vi "Ring下拉列表鼠标滚动事件.vi"(8 "error in (no error)":errorcluster caption="错误输入（无错误）", 9 "方向":enum16{"Horizontal", "Vertical"}(ring), 10 "Delta":i32, 11 "CtlRef":refnum<vi>) -> (0 "error out":errorcluster caption="错误输出", 3 "CtlRef 2":refnum<vi>)   [LabVIEW 2018]
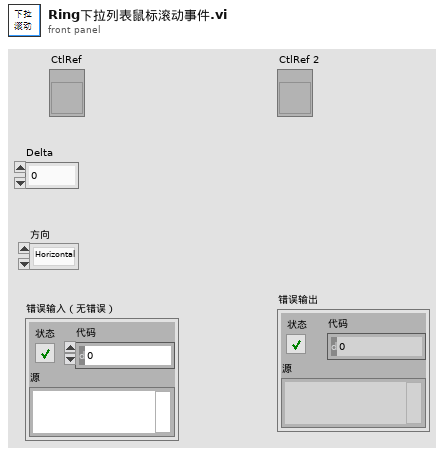
[diagram p1: front panel]
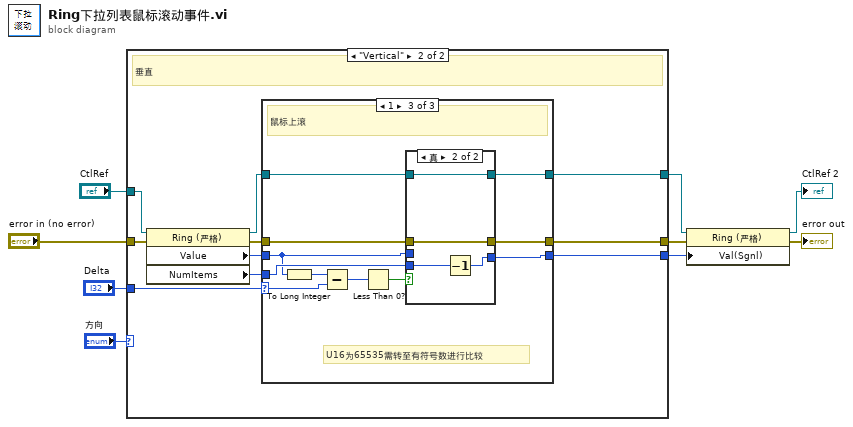
[diagram p0: block diagram]
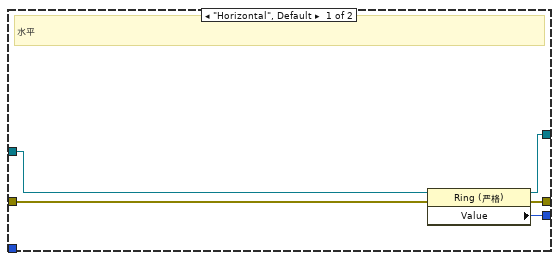
[diagram p2: hidden frame]
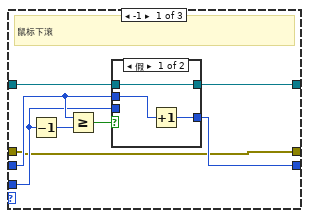
[diagram p3: hidden frame]
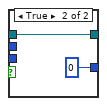
[diagram p4: hidden frame]
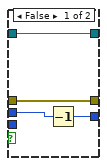
[diagram p6: hidden frame]
diagram:
  n1 = case shown="\"Vertical\"" "方向" {
    tunnel: "CtlRef" -> [w14 w24]
    tunnel: [w12 w21] -> w9
    tunnel: [w13 w20] -> w8
    tunnel: "Delta" -> [_ w18]
    tunnel: [w10 w17] -> w5
    tunnel: "error in (no error)" -> [w11 w15]
    frame "Horizontal", Default {
      # "水平"
      n2 = property class="Ring (严格)"(reference=w14, error in=w11) -> (reference out=w12:refnum<vi>, error out=w10:errorcluster, "Value"=w13:u16)
    }
    frame "Vertical" {
      # "垂直"
      n3 = property class="Ring (严格)"(reference=w24, error in=w15) -> (reference out=w23:refnum<vi>, error out=w16:errorcluster, "Value"=w22:u16, "NumItems"=w19:u32)
      n4 = case shown="1" w18 {
        selector: w18 -> [_ _ w46]
        tunnel: w23 -> [w27 w40 w49]
        tunnel: w22 -> [w29 w39 w47]
        tunnel: [w31 w40 w50] -> w21
        tunnel: [w30 w39 w51] -> w20
        tunnel: w19 -> [w28 _ w48]
        tunnel: [w25 w38 w42] -> w17
        tunnel: w16 -> [w25 w38 w41]
        frame -1 {
          # "鼠标下滚"
          n5 = Decrement(x=w28) -> (x-1=w26:u32)
          n6 = Greater Or Equal?(x=w29, y=w26) -> (x >= y?=w32:bool)
          n7 = case shown="假" w32 {
            tunnel: w29 -> [w35 _]
            tunnel: [w34 u16 0] -> w30
            tunnel: [w33 w36] -> w31
            tunnel: w28 -> [_ _]
            tunnel: w27 -> [w33 w36]
            frame False {
              n8 = Increment(x=w35) -> (x+1=w34:u16)
            }
            frame True {
            }
          }
        }
        frame 0, Default {
        }
        frame 1 {
          # "U16为65535需转至有符号数进行比较"
          # "鼠标上滚"
          n9 = To Long Integer(number=w47) -> (32bit integer=w43:i32)
          n10 = Subtract(x=w43, y=w46) -> (x-y=w44:i32)
          n11 = Less Than 0?(x=w44) -> (x < 0?=w45:bool)
          n12 = case shown="真" w45 {
            tunnel: w49 -> [w55 w59]
            tunnel: w47 -> [w54 _]
            tunnel: [w53 w58] -> w51
            tunnel: [w55 w59] -> w50
            tunnel: w48 -> [_ w57]
            tunnel: [w52 w56] -> w42
            tunnel: w41 -> [w52 w56]
            frame False {
              n13 = Decrement(x=w54) -> (x-1=w53:u16)
            }
            frame True {
              n14 = Decrement(x=w57) -> (x-1=w58:u32)
            }
          }
        }
      }
    }
  }
  n15 = property class="Ring (严格)"(reference=w9, error in=w5, "Val(Sgnl)"=w8) -> (reference out=→"CtlRef 2":refnum<vi>, error out=→"error out":errorcluster)
